vi "Get image date.vi"(8 "error in (no error)":errorcluster, 11 "CCDCamera in":refnum<class "Real Camera.lvclass">) -> (0 "error out":errorcluster, 3 "CCDCamera out":refnum<class "Real Camera.lvclass">)   [LabVIEW 2018, in "Real Camera.lvclass"]
doc: "Get the time stamp (in UTC) at the begining of the exposure"
uses:
  Real Camera.lvclass
  C:/Users/Denis/Desktop/S4ACS/S4ACS/Simulated_CCD_Camera/Simulated Camera.lvclass
  <vilib>/Utility/miscctls.llb/LVDateTimeRec.ctl
  Simulated_CCD_Camera/Simulated Camera.lvclass
panel:
  in  "date time rec":T1
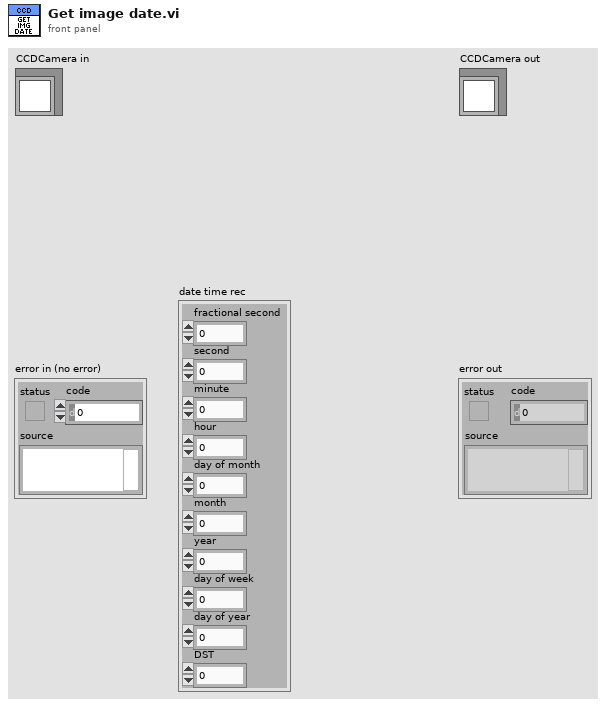
[diagram p1: front panel]
types:
  T1 = typedef "LVDateTimeRec.ctl" = cluster{"fractional second":dbl, "second":i32, "minute":i32, "hour":i32, "day of month":i32, "month":i32, "year":i32, "day of week":i32, "day of year":i32, "DST":i32}
  T2 = cluster{"CYCLES_DONE":u16, "LAST_IMAGE_NAME":string, "USED_DISK_SPACE":u16, "FRAMES_DONE":u16, "CCD_STATUS":string, "CURRENT_TEMPERATURE":i16, "TEMPERATURE_STATUS":string, "FRAME_EXPOSURE_TIME":sgl, "ERROR":bool, "SERIAL_NUMBER":u16, "ACQUIRING":bool, "IMAGE_INDEX":u32, "SEQS_DONE":u16, "ACS MODE":bool}
  T3 = typedef "SYSTEMTIME structure typedef.ctl" = cluster{"Year":u16, "Month":u16, "DayOfWeek":u16, "Date":u16, "Hour":u16, "Minute":u16, "Second":u16, "Milliseconds":u16}
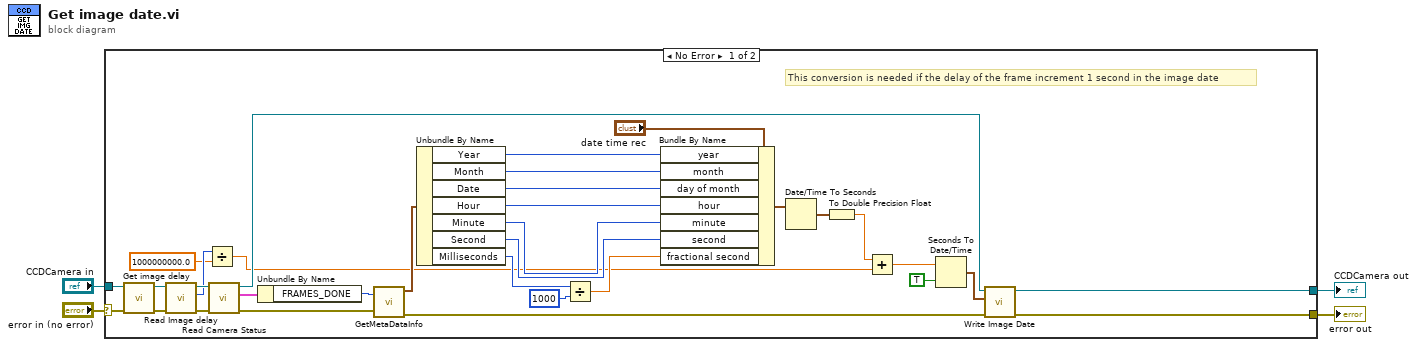
[diagram p0: block diagram]
diagram:
  n1 = case shown="No Error" "error in (no error)" {
    selector: "error in (no error)" -> [w14 w38]
    tunnel: [w36 w38] -> w3
    tunnel: "CCDCamera in" -> [w13 w39]
    tunnel: [w35 w39] -> w1
    frame No Error {
      # "This conversion is needed if the delay of the frame increment 1 second in the image date"
      n2 = call-dynamic "Get image delay.vi"("error in (no error)"=w14, "CCDCamera in"=w13) -> ("error out"=w12:errorcluster, "CCDCamera out"=w9:refnum<class "Real Camera.lvclass">)  [unwired: 8 in]
      n3 = call-dynamic "Read Image delay.vi"("error in (no error)"=w12, "Simulated_CCD_Camera in"=w9) -> ("error out"=w11:errorcluster, "Image delay"=w8:u64, "Simulated_CCD_Camera out"=w10:refnum<class "Real Camera.lvclass">)  [unwired: 7 in]
      n4 = Divide(x=w8, y=1000000000.0) -> (x/y=w6:dbl)
      n5 = call "Read Camera Status.vi"("error in (no error)"=w11, "CCDCamera in"=w10) -> ("error out"=w33:errorcluster, "Camera Status"=w34:T2, "CCDCamera out"=w32:refnum<class "Real Camera.lvclass">)  [unwired: 7 in]
      n6 = Unbundle By Name(w34) -> ("FRAMES_DONE"=w15:u16)
      n7 = call <userlib>:"GetMetaDataInfo.vi"("index"=w15, "error in (no error)"=w33) -> ("SYSTEMTIME"=w17:T3, "error out"=w37:errorcluster)  [unwired: 2 out]
      n8 = Unbundle By Name(w17) -> ("Year"=w24:u16, "Month"=w23:u16, "Date"=w22:u16, "Hour"=w21:u16, "Minute"=w20:u16, "Second"=w19:u16, "Milliseconds"=w26:u16)
      n9 = Divide(x=w26, y=1000) -> (x/y=w18:dbl)
      n10 = Bundle By Name(cluster="date time rec", "year"=w24, "month"=w23, "day of month"=w22, "hour"=w21, "minute"=w20, "second"=w19, "fractional second"=w18) -> (w30:T1)
      n11 = Date/Time To Seconds(2:w30) -> (0:w29:timestamp)  [unwired: 1 in]
      n12 = To Double Precision Float(number=w29) -> (double precision float=w28:dbl)
      n13 = Add(x=w28, y=w6) -> (x+y=w27:dbl)
      n14 = Seconds To Date/Time(time stamp (now)=w27, to UTC (F)=TRUE) -> (date time rec=w5:T1)
      n15 = call-dynamic "Write Image Date.vi"("error in (no error)"=w37, "SYSTEMTIME"=w5, "Simulated_CCD_Camera in"=w32) -> ("error out"=w36:errorcluster, "Simulated_CCD_Camera out"=w35:refnum<class "Real Camera.lvclass">)  [unwired: 7 in]
    }
    frame Error {
    }
  }
  "error out" <- w3
  "CCDCamera out" <- w1
